vi "Get Enum Arm Positions.vi"(0 "Previous Arm Position":T1, 5 "Pick-up Button":bool, 7 "Shoot Button":bool, 9 "Truss Button":bool, 11 "Idle Button":bool, 12 "Manual Button":bool) -> (6 "New Arm Position":T1)   [LabVIEW 2013]
uses:
  Arm Postions Enum Typedef.ctl
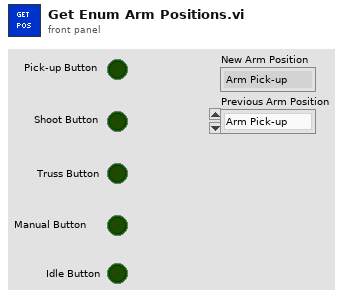
[diagram p1: front panel]
types:
  T1 = typedef "Arm Postions Enum Typedef.ctl" = enum16{"Arm Pick-up", "Idle", "Arm Shoot", "Arm Truss", "Manual"}
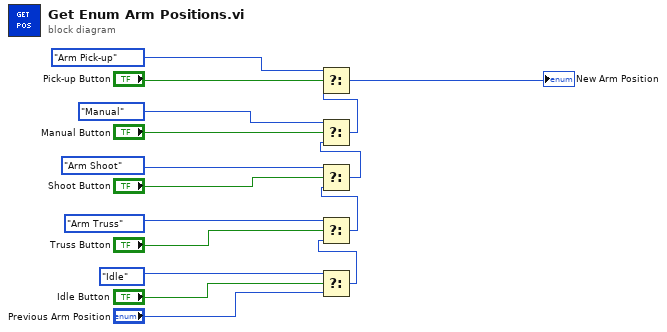
[diagram p0: block diagram]
diagram:
  n1 = Select(t=Arm_Postions_Enum_Typedef."Idle" ("Arm Command.Arm Positions"), s="Idle Button", f="Previous Arm Position") -> (s? t:f=w2:T1)
  n2 = Select(t=Arm_Postions_Enum_Typedef."Arm Truss" ("Arm Command.Arm Positions"), s="Truss Button", f=w2) -> (s? t:f=w16:T1)
  n3 = Select(t=Arm_Postions_Enum_Typedef."Arm Shoot" ("Arm Command.Arm Positions"), s="Shoot Button", f=w16) -> (s? t:f=w15:T1)
  n4 = Select(t=Arm_Postions_Enum_Typedef."Manual" ("Arm Command.Arm Positions"), s="Manual Button", f=w15) -> (s? t:f=w14:T1)
  n5 = Select(t=Arm_Postions_Enum_Typedef."Arm Pick-up" ("Arm Command.Arm Positions"), s="Pick-up Button", f=w14) -> (s? t:f=→"New Arm Position":T1)
